vi "Write num_to_remove.vi"(8 "error in (no error)":errorcluster, 10 "num_to_remove":u64, 11 "Remove Log Message MSG in":refnum<class "Remove Log Message MSG.lvclass">) -> (0 "error out":errorcluster, 3 "Remove Log Message MSG out":refnum<class "Remove Log Message MSG.lvclass">)   [LabVIEW 2016, in "Controller.lvlib" / "Remove Log Message MSG.lvclass"]
uses:
  Remove Log Message MSG.lvclass
  Remove Log Message MSG.lvclass/Remove Log Message MSG.ctl
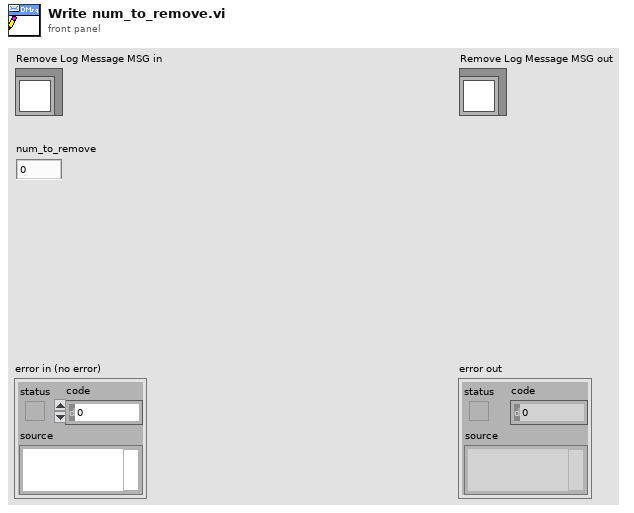
[diagram p1: front panel]
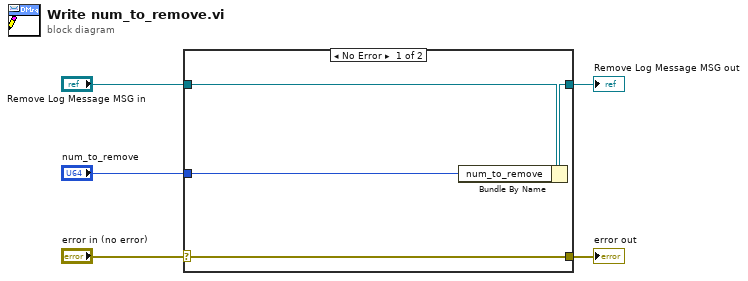
[diagram p0: block diagram]
diagram:
  n1 = case shown="No Error" "error in (no error)" {
    selector: "error in (no error)" -> [w9 w10]
    tunnel: [w9 w10] -> w4
    tunnel: [w7 w11] -> w2
    tunnel: "Remove Log Message MSG in" -> [w8 w11]
    tunnel: "num_to_remove" -> [w6 _]
    frame No Error {
      n2 = Bundle By Name(cluster=w8, "num_to_remove"=w6) -> (w7:refnum<class "Remove Log Message MSG.lvclass">)
    }
    frame Error {
    }
  }
  "error out" <- w4
  "Remove Log Message MSG out" <- w2
